vi "Log Space.vi"(8 "error in (no error)":errorcluster, 9 "Number of Samples":u32, 10 "Maximum":dbl, 11 "Minimum":dbl) -> (0 "error out":errorcluster, 3 "Array":dbl[](array[numeric]))   [LabVIEW 2013]
doc: "This subVI will create an logarithmically spaced array of elements equal to the Number of Samples between the Minimum and Maximum.\n\nImportant: The Minimum and maximum are formatted as powers of ten, so a Minimum of -1 and a Maximum of 9 gives an array between 0.1 and 1,000,000,000."
panel:
  # "Overview: Use this VI to create an logarithmically spaced array of elements equal to the Number of Samples between the Minimum and Maximum.\nPay Attention :The Minimum and maximum are formatted as powers of ten, so a Minimum of -1 and a Maximum of 9 gives an array between 0.1 and 1,000,000,000.\nRequirements: LabVIEW 2012\nInstructions:\n1. Set Parameters (Min Max and # of samples)\n2. Run VI"
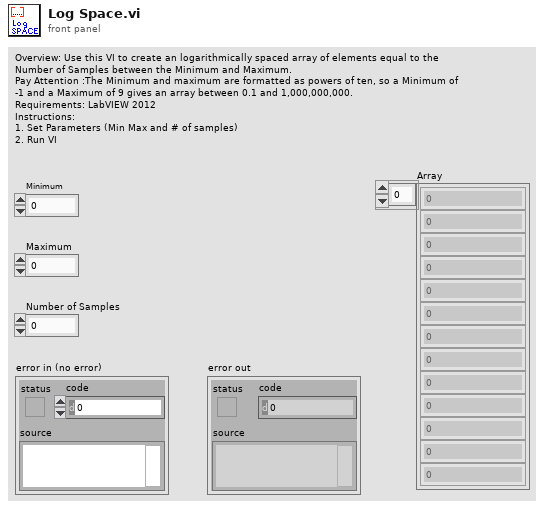
[diagram p1: front panel]
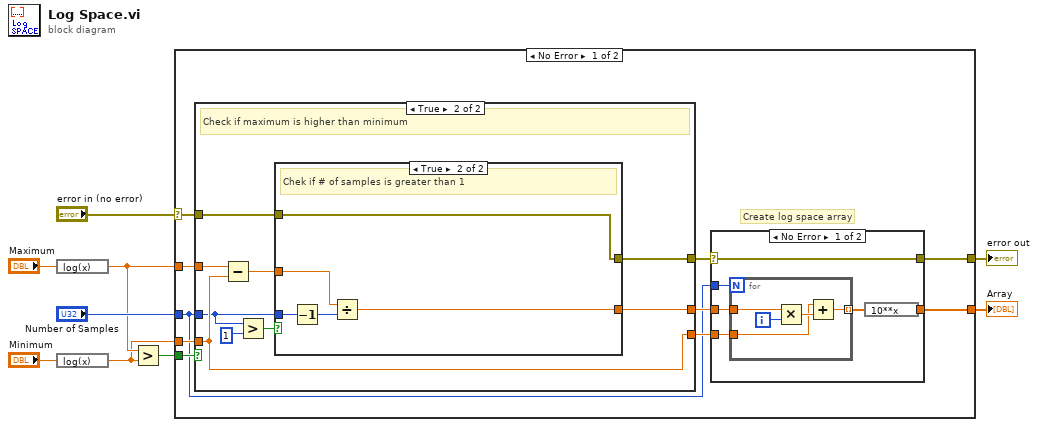
[diagram p0: block diagram]
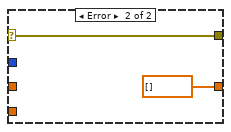
[diagram p2: hidden frame]
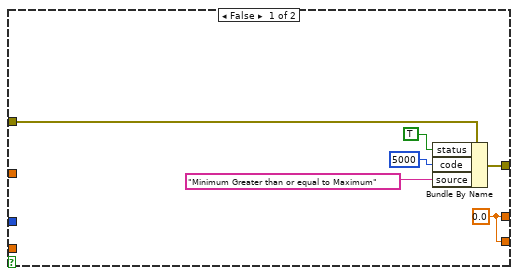
[diagram p3: hidden frame]
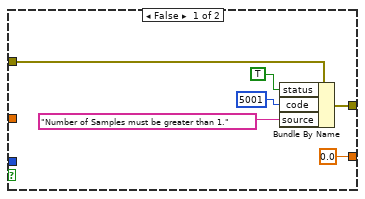
[diagram p4: hidden frame]
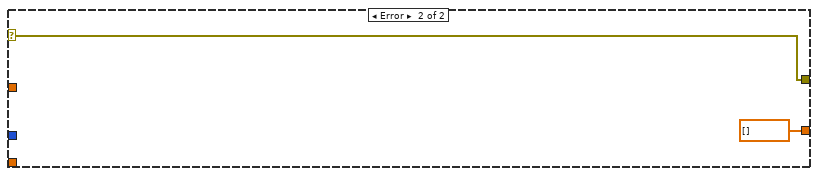
[diagram p5: hidden frame]
diagram:
  n1 = expression code="log(x)"("Maximum") -> (w3:dbl)
  n2 = expression code="log(x)"("Minimum") -> (w1:dbl)
  n3 = Greater?(x=w3, y=w1) -> (0:w9:bool)
  n4 = case shown="No Error" "error in (no error)" {
    selector: "error in (no error)" -> [w11 w59]
    tunnel: w9 -> [w19 _]
    tunnel: w3 -> [w18 _]
    tunnel: w1 -> [w17 _]
    tunnel: [w15 w59] -> w7
    tunnel: "Number of Samples" -> [w12 _]
    tunnel: [w10 dbl[] []] -> w5
    frame No Error {
      # "Create log space array"
      n5 = case shown="True" w19 {
        tunnel: w11 -> [w38 w45]
        tunnel: [w34 w44] -> w16
        tunnel: w18 -> [_ w39]
        tunnel: w17 -> [_ w43]
        tunnel: w12 -> [_ w40]
        tunnel: [w33 w46] -> w14
        tunnel: [w33 w43] -> w13
        frame False {
          w33 = 0.0
          n6 = Bundle By Name(cluster=w38, "status"=TRUE, "code"=5000, "source"="Minimum Greater than or equal to Maximum") -> (w34:errorcluster)
        }
        frame True {
          # "Check if maximum is higher than minimum"
          n7 = Subtract(x=w39, y=w43) -> (x-y=w47:dbl)
          n8 = Greater?(x=w40, y=u32 1) -> (0:w41:bool)
          n9 = case shown="True" w41 {
            tunnel: w47 -> [_ w58]
            tunnel: [0.0 w57] -> w46
            tunnel: w45 -> [w52 w56]
            tunnel: [w51 w56] -> w44
            tunnel: w40 -> [_ w54]
            frame False {
              n10 = Bundle By Name(cluster=w52, "status"=TRUE, "code"=5001, "source"="Number of Samples must be greater than 1.") -> (w51:errorcluster)
            }
            frame True {
              # "Chek if # of samples is greater than 1"
              n11 = Decrement(x=w54) -> (x-1=w55:u32)
              n12 = Divide(x=w58, y=w55) -> (x/y=w57:dbl)
            }
          }
        }
      }
      n13 = case shown="No Error" w16 {
        selector: w16 -> [w25 w31]
        tunnel: [w25 w31] -> w15
        tunnel: w14 -> [w22 _]
        tunnel: w13 -> [w23 _]
        tunnel: w12 -> [w24 _]
        tunnel: [w20 dbl[] []] -> w10
        frame No Error {
          n14 = for {
            N: w24 -> [_]
            tunnel: w23 -> [w27]
            tunnel: w22 -> [w29]
            tunnel: [w26] -> w21 mode=indexing
            i -> [w30]
            n15 = Multiply(x=w29, y=w30) -> (x*y=w28:dbl)
            n16 = Add(x=w27, y=w28) -> (x+y=w26:dbl)
          }
          n17 = expression code="10**x"(w21) -> (w20:dbl[])
        }
        frame Error {
        }
      }
    }
    frame Error {
    }
  }
  "error out" <- w7
  "Array" <- w5
